vi "FestoCPX.DO.Write.vi"(8 "error in (no error)":errorcluster, 11 "TCP Conn Ref":refnum<k5>) -> (0 "error out":errorcluster, 1 "changed?":bool, 3 "TCP Conn Ref out":refnum<k5>)   [LabVIEW 2016]
uses:
  FestoCPX.DO.Data.Fglb.Action.ctl
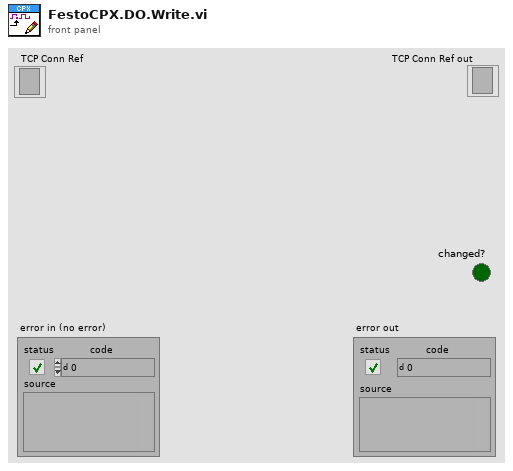
[diagram p1: front panel]
types:
  T1 = typedef "FestoCPX.DO.Data.Fglb.Action.ctl" = enum16{"init", "set", "get", "check", "select", "reset"}
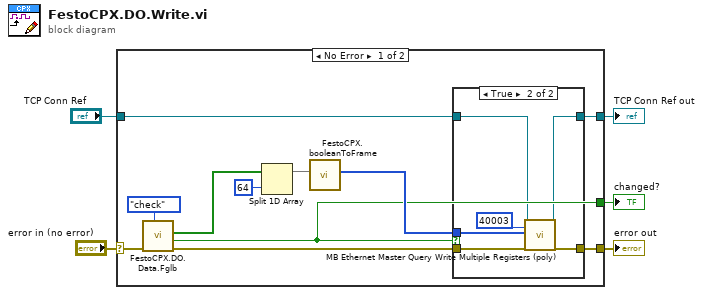
[diagram p0: block diagram]
diagram:
  n1 = case shown="No Error" "error in (no error)" {
    selector: "error in (no error)" -> [w12 w25]
    tunnel: "TCP Conn Ref" -> [w14 w26]
    tunnel: [w15 w26] -> w4
    tunnel: [w16 w25] -> w2
    tunnel: [w6 _] -> w1
    frame No Error {
      n2 = call "FestoCPX.DO.Data.Fglb.vi"("state (get all)"=FestoCPX.DO.Data.Fglb.Action."check", "error in (no error)"=w12) -> ("error out"=w8:errorcluster, "changed?"=w6:bool, "State out"=w10:bool[])  [unwired: 7 in]
      n3 = Split 1D Array(array=w10, index=64) -> (first subarray=w9:bool[])  [unwired: 1 out]
      n4 = call "FestoCPX.booleanToFrame.vi"("Raw Array"=w9) -> ("Bytes DO"=w7:u16[])  [unwired: 10 in]
      n5 = case shown="True" w6 {
        tunnel: [w17 w24] -> w16
        tunnel: [w18 w22] -> w15
        tunnel: w14 -> [w18 w21]
        tunnel: w8 -> [w17 w20]
        tunnel: w7 -> [_ w19]
        frame False {
        }
        frame True {
          n6 = call "MB Ethernet Master Query Write Multiple Registers (poly).vi"("TCP Connection Refnum in"=w21, "Starting Address"=u16 40003, "Registers"=w19, "error in"=w20) -> ("TCP Connection Refnum (dup)"=w22:refnum<k5>, "error out"=w24:errorcluster)  [unwired: 13 in, 1 out]
        }
      }
    }
    frame Error {
    }
  }
  "error out" <- w2
  "TCP Conn Ref out" <- w4
  "changed?" <- w1
